vi "Export serials.vi"(8 "error in (no error)":errorcluster, 11 "REF":T1) -> (0 "error out":errorcluster, 2 "Success?":bool, 3 "REF OUT":T1)   [LabVIEW 2024]
uses:
  CTRLS/REF.ctl
  CTRLS/Main Tabs.ctl
  CTRLS/Open Batch Data.ctl
  CTRLS/DM_Data.ctl
  CTRLS/run statistics.ctl
  CTRLS/System settings.ctl
  CTRLS/Printer Message settings.ctl
  CTRLS/Serials DB Operations Enum.ctl
  <vilib>/Utility/file.llb/Write Delimited Spreadsheet (string).vi
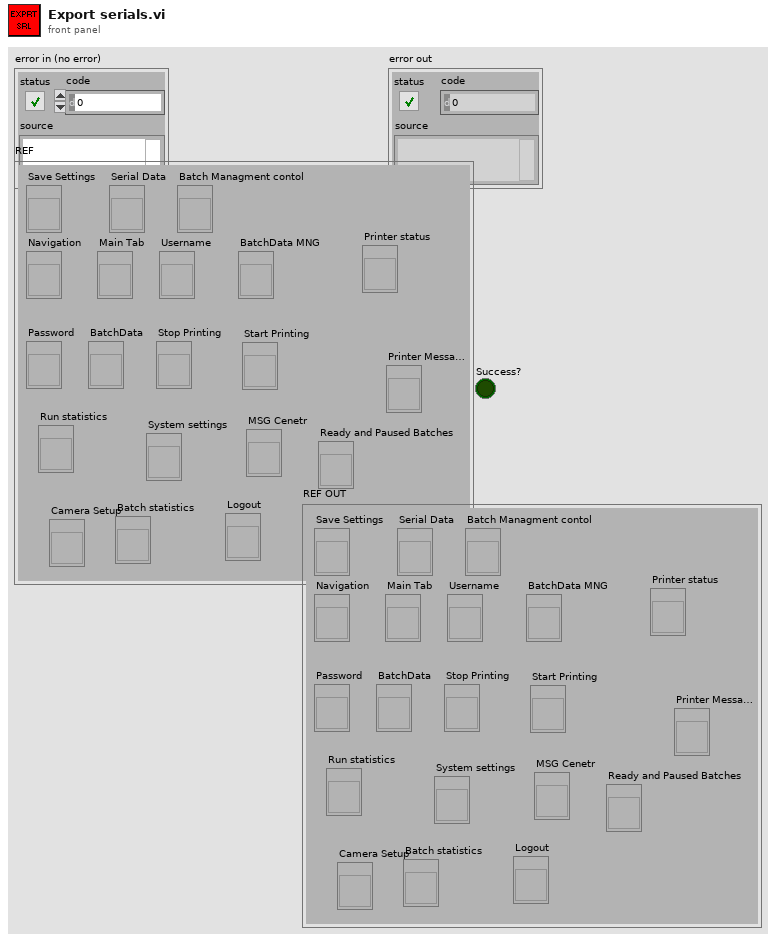
[diagram p1: front panel]
types:
  T1 = typedef "REF.ctl" = cluster{"Save Settings":refnum<vi>, "Navigation":refnum<vi>, "Main Tab":refnum<vi>, "Password":refnum<vi>, "BatchData":refnum<vi>, "Serial Data":refnum<vi>, "Username":refnum<vi>, "Stop Printing":refnum<vi>, "Run statistics":refnum<vi>, "System settings":refnum<vi>, "Batch Managment contol":refnum<vi>, "Start Printing":refnum<vi>, "BatchData MNG":refnum<vi>, "MSG Cenetr":refnum<vi>, "Printer status":refnum<vi>, "Printer Message Config":refnum<vi>, "Ready and Paused Batches":refnum<vi>, "Camera Setup":refnum<vi>, "Batch statistics":refnum<vi>, "Logout":refnum<vi>}
  T2 = typedef "Serials DB Operations Enum.ctl" = enum16{"Update serial verify status", "Get serials Based on Status", "Insert serials", "Update serial print status", "Get all Batch Serials", "Get Serial Status"}
  T3 = typedef "System settings.ctl" = cluster{"Machine IP":string, "Camera IP":string, "Printer IP":string, "Scanner settings":string, "Server Path":path, "Sending Port":u32, "Recieveing Port":u32}
  T4 = typedef "Open Batch Data.ctl" = cluster{"Batch Name":string, "Batch Number":string, "GTIN":string, "Expiry Date":string, "MFG Date":string}
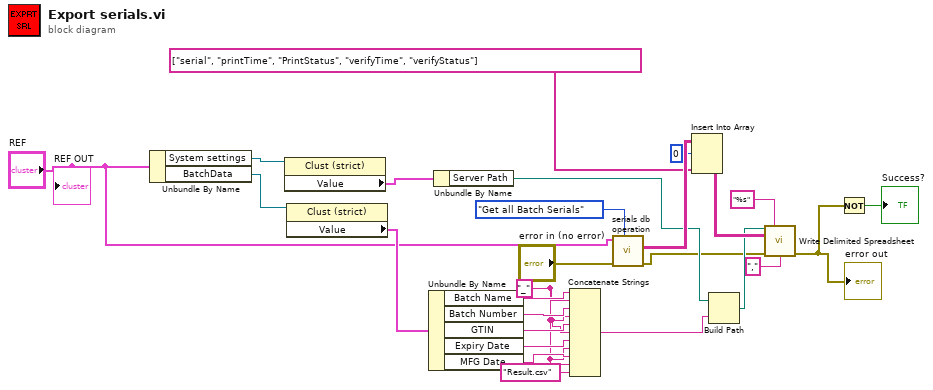
[diagram p0: block diagram]
diagram:
  w10 = "_" ("string")
  n1 = Unbundle By Name("REF") -> ("System settings"=w26:refnum<vi>, "BatchData"=w24:refnum<vi>)
  n2 = property class="Clust (strict)"(reference=w26) -> ("Value"=w25:T3)  [unwired: 1 in, 2 out]
  n3 = property class="Clust (strict)"(reference=w24) -> ("Value"=w16:T4)  [unwired: 1 in, 2 out]
  n4 = Unbundle By Name(w16) -> ("Batch Name"=w15:string, "Batch Number"=w14:string, "GTIN"=w13:string, "Expiry Date"=w12:string, "MFG Date"=w11:string)
  n5 = Unbundle By Name(w25) -> ("Server Path"=w8:path)
  n6 = Concatenate Strings(w15, w10, w14, w10, w13, w10, w12, w10, w11, w10, "Result.csv" ("string")) -> (w7:string)
  n7 = call "serials db operation.vi"("SRL DB OP"=Serials_DB_Operations_Enum."Get all Batch Serials", "error in (no error)"="error in (no error)", "REF"="REF") -> ("error out"=w5:errorcluster, "Fetched Serials"=w20:string[][])  [unwired: 5 in, 2 out]
  n8 = Insert Into Array(array=w20, index (row)=0, new element=string[] ["serial", "printTime", "PrintStatus", "verifyTime", "verifyStatus"] ("new element/subarray")) -> (w17:string[][])  [unwired: 1 in]
  n9 = Build Path(base path=w8, name or relative path=w7) -> (appended path=w6:path)
  n10 = call-poly <vilib>:"Write Delimited Spreadsheet.vi"("file path (dialog if empty)"=w6, "format (%s)"="%s" ("format (%.3f)"), "2D data"=w17, "error in (no error)"=w5, "delimiter (\\t)"="," ("delimiter (\\t)")) -> ("error out"=w2:errorcluster)  [unwired: 9 in, 1 out]
  "error out" <- w2
  n11 = Not(x=w2) -> (.not. x?=→"Success?":bool)
  "REF OUT" <- "REF"
